vi "Init M3102A.vi"(8 "errorIn":errorcluster) -> (0 "errorOut":errorcluster, 3 "moduleID":i32)   [LabVIEW 2021]
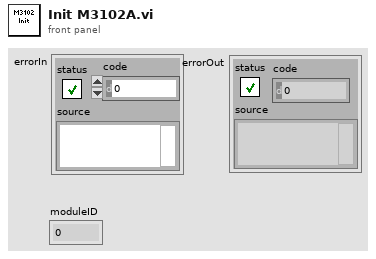
[diagram p1: front panel]
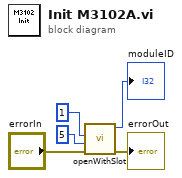
[diagram p0: block diagram]
diagram:
  n1 = call <vilib>:"openWithSlot.vi"("errorIn"="errorIn", "nSlot"=5, "nChassis"=1) -> ("errorOut"=→"errorOut":errorcluster, "moduleID"=→"moduleID":i32)  [unwired: 3 in]
